vi "background.vi"() -> ()   [LabVIEW 8.6]
panel:
  out "result string":string
  out "function return":string
  out "error out":errorcluster
  out "function return 2":string
  # "background.xlsx"
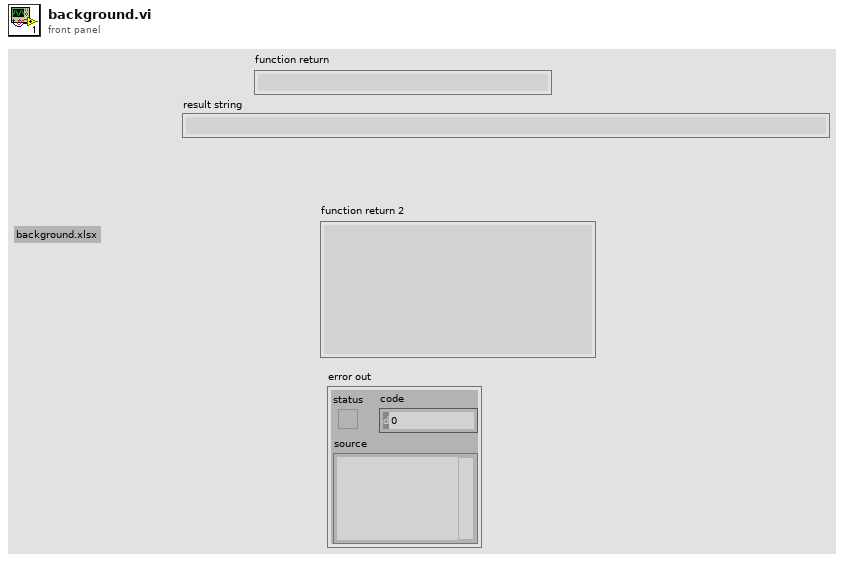
[diagram p1: front panel]
types:
  T1 = enum32{"invalid app kind", "Development System", "Run Time System", "Student Edition", "Embedded LabVIEW", "Evaluation", "Custom"}
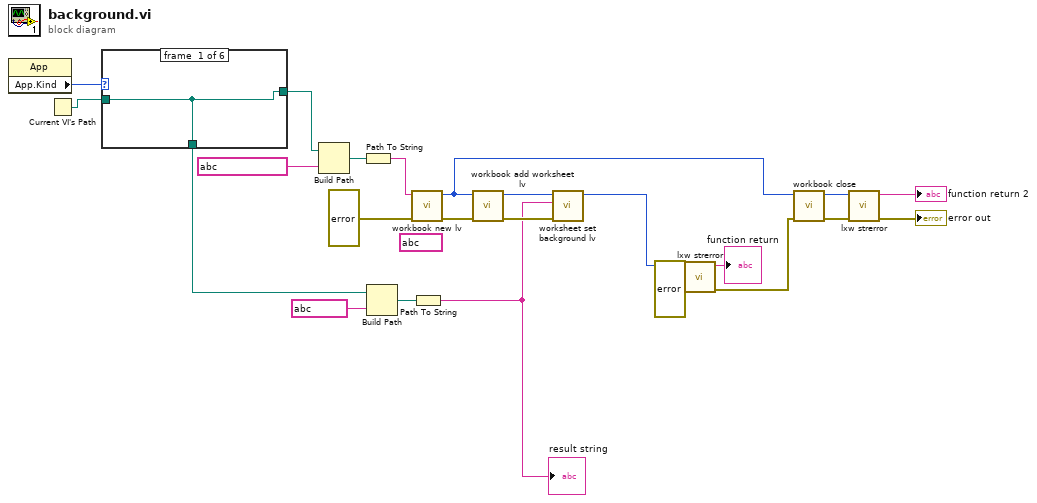
[diagram p0: block diagram]
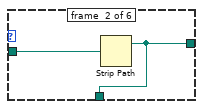
[diagram p2: hidden frame]
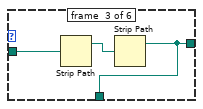
[diagram p3: hidden frame]
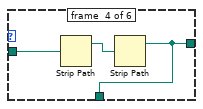
[diagram p4: hidden frame]
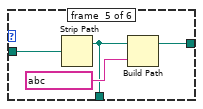
[diagram p5: hidden frame]
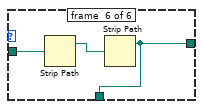
[diagram p6: hidden frame]
diagram:
  (unwired) string ? ("sheetname")
  n1 = property class="App"() -> ("App.Kind"=w23:T1)  [unwired: 2 in, 2 out]
  n2 = Current VI's Path() -> (path=w22:path)
  n3 = case shown="\"Evaluation\"" w23 {
    tunnel: w22 -> [w24 w26 w29 w32 w36 w39]
    tunnel: [w24 w25 w27 w30 w35 w37] -> w21
    tunnel: [w24 w25 w27 w30 w33 w37] -> w7
    frame #0 {
    }
    frame #1 {
      n4 = Strip Path(path=w26) -> (stripped path=w25:path)  [unwired: 1 out]
    }
    frame #2 {
      n5 = Strip Path(path=w29) -> (stripped path=w28:path)  [unwired: 1 out]
      n6 = Strip Path(path=w28) -> (stripped path=w27:path)  [unwired: 1 out]
    }
    frame #3 {
      n7 = Strip Path(path=w32) -> (stripped path=w31:path)  [unwired: 1 out]
      n8 = Strip Path(path=w31) -> (stripped path=w30:path)  [unwired: 1 out]
    }
    frame #4 {
      n9 = Strip Path(path=w36) -> (stripped path=w33:path)  [unwired: 1 out]
      n10 = Build Path(base path=w33, name or relative path=string ?) -> (appended path=w35:path)
    }
    frame #5 {
      n11 = Strip Path(path=w39) -> (stripped path=w38:path)  [unwired: 1 out]
      n12 = Strip Path(path=w38) -> (stripped path=w37:path)  [unwired: 1 out]
    }
  }
  n13 = Build Path(base path=w21, name or relative path=string ? ("filename")) -> (appended path=w12:path)
  n14 = Path To String(path=w12) -> (string=w11:string)
  n15 = Build Path(base path=w7, name or relative path=string ? ("filename")) -> (appended path=w4:path)
  n16 = call "workbook new lv.vi"("error in (no error)"=errorcluster ?, "filename"=w11) -> ("error out"=w19:errorcluster, "function return"=w13:u32)  [unwired: 8 in]
  n17 = Path To String(path=w4) -> (string=w1:string)
  "result string" <- w1
  n18 = call "workbook add worksheet lv.vi"("error in (no error)"=w19, "workbook"=w13) -> ("error out"=w2:errorcluster, "function return"=w5:u32)  [unwired: 8 in]
  n19 = call "worksheet set background lv.vi"("error in (no error)"=w2, "filename"=w1, "worksheet"=w5) -> ("function return"=w3:u32)  [unwired: 7 in, 1 out]
  n20 = call "lxw strerror.vi"("error in (no error)"=errorcluster ?, "error_num"=w3) -> ("error out"=w8:errorcluster, "function return"=→"function return":string)  [unwired: 8 in]
  n21 = call "workbook close.vi"("error in (no error)"=w8, "workbook"=w13) -> ("error out"=w15:errorcluster, "function return"=w17:u32)  [unwired: 8 in]
  n22 = call "lxw strerror.vi"("error in (no error)"=w15, "error_num"=w17) -> ("error out"=→"error out":errorcluster, "function return"=→"function return 2":string)  [unwired: 8 in]
